vi "Config Dir Path.vi"() -> (3 "App.Dir":path)   [LabVIEW 2010, in "MonitorServer.lvlib"]
uses:
  MonitorServer.lvlib
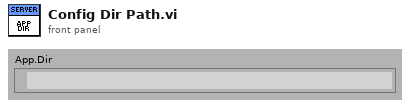
[diagram p1: front panel]
types:
  T1 = enum32{"invalid app kind", "Development System", "Run Time System", "Student Edition", "Embedded LabVIEW", "Evaluation", "Custom"}
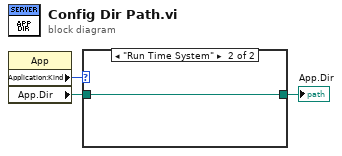
[diagram p0: block diagram]
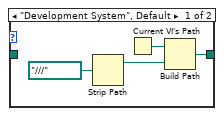
[diagram p2: hidden frame]
diagram:
  n1 = property class="App"() -> ("Application:Kind"=w2:T1, "App.Dir"=w3:path)  [unwired: 2 in, 2 out]
  n2 = case shown="\"Run Time System\"" w2 {
    tunnel: [w7 w8] -> w1
    tunnel: w3 -> [_ w8]
    frame "Development System", Default {
      n3 = Strip Path(path=path "../../../.." ("relative path (.)")) -> (stripped path=w6:path)  [unwired: 1 out]
      n4 = Current VI's Path() -> (path=w5:path)
      n5 = Build Path(base path=w5, name or relative path=w6) -> (appended path=w7:path)
    }
    frame "Run Time System" {
    }
  }
  "App.Dir" <- w1
